vi "Get Molecular Density.vi"(1 "thermoCond":cluster{"T (degC)":dbl, "P (mb)":dbl}) -> (0 "M (m-3)":dbl)   [LabVIEW 2019, in "Atmospheric Library.lvlib"]
doc: "Returns the molecular number density as a function of temperature and pressure based on the ideal gas law."
uses:
  Atmospheric Library.lvlib
  Atmospheric Constants.vi
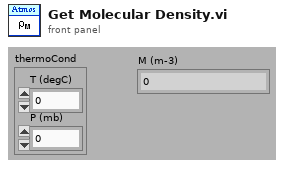
[diagram p1: front panel]
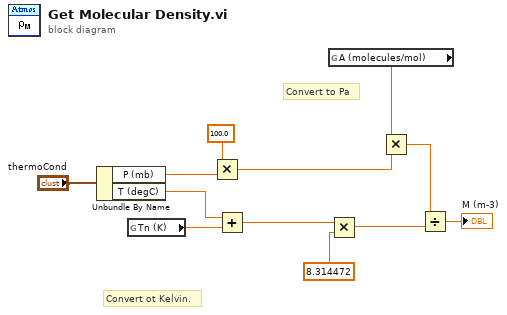
[diagram p0: block diagram]
diagram:
  # "Convert ot Kelvin."
  # "Convert to Pa"
  n1 = Unbundle By Name("thermoCond") -> ("P (mb)"=w8:dbl, "T (degC)"=w5:dbl)
  n2 = global read "Atmospheric Constants.vi" "Tn (K)"() -> (w7:dbl)
  n3 = Multiply(x=100.0 ("y"), y=w8) -> (x*y=w3:dbl)
  n4 = Add(x=w5, y=w7) -> (x+y=w10:dbl)
  n5 = global read "Atmospheric Constants.vi" "A (molecules/mol)"() -> (w4:dbl)
  n6 = Multiply(x=w10, y=8.314472 ("R (J/(mol K)")) -> (x*y=w11:dbl)
  n7 = Multiply(x=w4, y=w3) -> (x*y=w2:dbl)
  n8 = Divide(x=w2, y=w11) -> (x/y=→"M (m-3)":dbl)
